vi "standard frame scan geometry_MD.vi"() -> (3 "frame scan geometry out":waveform(dbl)[](array[waveform]))   [LabVIEW 2012]
uses:
  GFG/GFGnumericGet.vi
  GFG/GFGbooleanGet.vi
  <vilib>/Analysis/coordinate.llb/2D Cartesian Coordinate Rotation (Array).vi
  GFG/GFG library.lvlib
  <vilib>/Analysis/NI_AALPro.lvlib
panel:
  out "x waveform":waveform(dbl)
  out "y waveform":waveform(dbl)
  out "Waveform Graph 2":waveform(dbl)(graph)
  out "Waveform Graph":waveform(dbl)(graph)
  out "y waveform (two frames)":dbl[](array[numeric])
  out "x waveform (two frames)":dbl[](array[numeric])
  out "XY Graph":cluster{"Y":dbl[], "Y":dbl[]}[](graph)
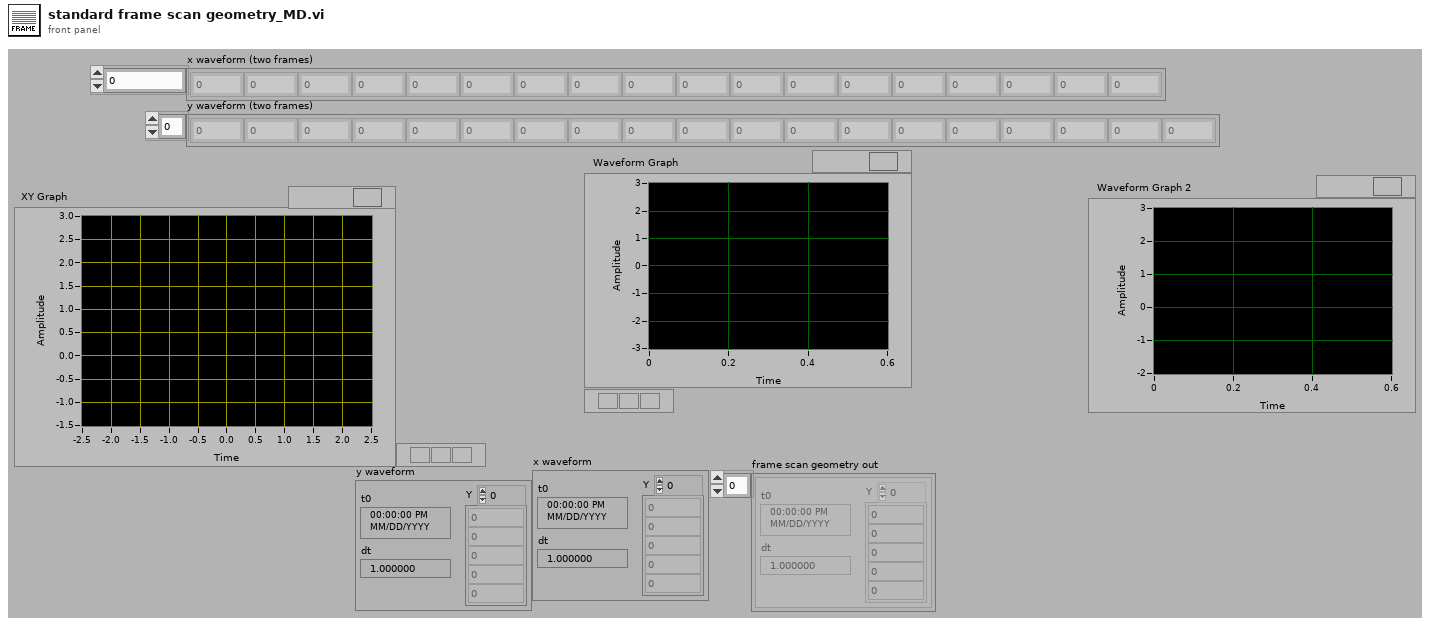
[diagram p1: front panel]
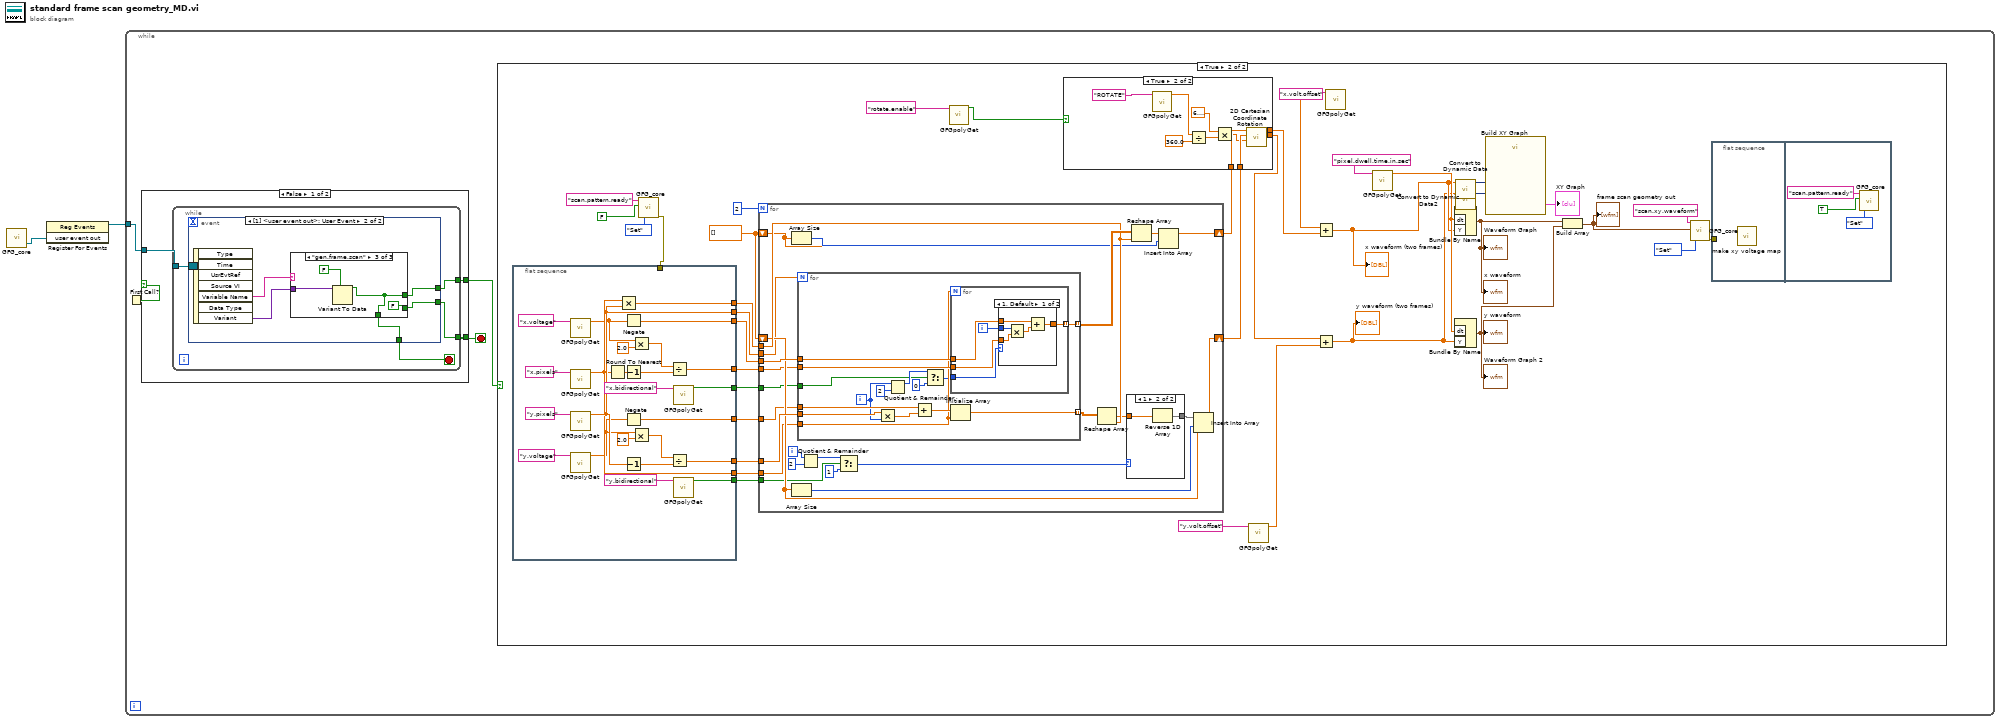
[diagram p0: block diagram]
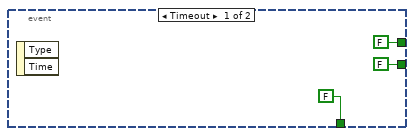
[diagram p2: hidden frame]
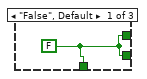
[diagram p3: hidden frame]
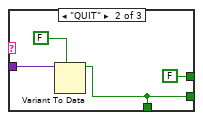
[diagram p4: hidden frame]
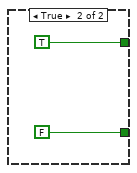
[diagram p5: hidden frame]
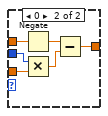
[diagram p9: hidden frame]
diagram:
  n1 = call "GFG_core.vi"() -> ("user event out"=w2:refnum<user-event>)  [unwired: 13 in, 6 out]
  n2 = register-events(w2) -> (reference out=w1:refnum<event-registration>)  [unwired: 2 in, 1 out]
  n3 = while {
    tunnel: w1 -> [w6]
    stop <- w5 stop-if-true
    n4 = First Call?() -> (First Call?: T/F=w3:bool)
    n5 = case shown="False" w3 {
      tunnel: w6 -> [w9 _]
      tunnel: [w8 FALSE ("NewVal")] -> w5
      tunnel: [w7 TRUE ("NewVal")] -> w4
      frame False {
        n6 = while {
          tunnel: w9 -> [w13]
          tunnel: [w11] -> w8
          tunnel: [w12] -> w7
          stop <- w10 stop-if-true
          n7 = event shown="[1] <user event out>: User Event" {
            selector: w13 -> [_ _]
            dyn-events: _ -> [_ _]
            timeout: _ -> [_ _]
            tunnel: [FALSE ("NewVal") w20] -> w12
            tunnel: [FALSE ("NewVal") w19] -> w11
            tunnel: [FALSE w17] -> w10
            event Timeout {
              n8 = event-data() -> ()  [unwired: 1 in, 2 out]
            }
            event User Event {
              n9 = event-data() -> ("Variable Name"=w21:string, "Variant"=w18:variant)  [unwired: 1 in, 5 out]
              n10 = case shown="\"gen.frame.scan\"" w21 {
                tunnel: [w22 FALSE ("NewVal") w27] -> w20
                tunnel: [w22 w23 FALSE] -> w19
                tunnel: w18 -> [_ w26 w28]
                tunnel: [w22 w23 w27] -> w17
                frame "False", Default {
                  w22 = FALSE ("NewVal")
                }
                frame "QUIT" {
                  n11 = Variant To Data(type=FALSE ("NewVal"), Variant=w26) -> (data=w23:bool)  [unwired: 1 in, 1 out]
                }
                frame "gen.frame.scan" {
                  n12 = Variant To Data(type=FALSE ("NewVal"), Variant=w28) -> (data=w27:bool)  [unwired: 1 in, 1 out]
                }
              }
            }
          }
        }
      }
      frame True {
      }
    }
    n13 = case shown="True" w4 {
      frame False {
      }
      frame True {
        w64 = dbl[] []
        n14 = flat-sequence {
          tunnel: [w92] -> w70
          tunnel: [w91] -> w69
          tunnel: [w89] -> w63
          tunnel: [w85] -> w62
          tunnel: [w84] -> w61
          tunnel: [w83] -> w60
          tunnel: [w81] -> w59
          tunnel: [w75] -> w58
          tunnel: [w73] -> w57
          tunnel: w33 -> [_]
          frame #0 {
            n15 = call-poly "GFGpolyGet.vi"("Variable Name in"="x.voltage" ("Tag in")) -> ("Numeric"=w79:dbl)  [unwired: 9 in, 1 out]
            n16 = call-poly "GFGpolyGet.vi"("Variable Name in"="x.pixels" ("Tag in")) -> ("Numeric"=w81:dbl)  [unwired: 9 in, 1 out]
            n17 = call-poly "GFGpolyGet.vi"("Variable Name in"="y.pixels" ("Tag in")) -> ("Numeric"=w83:dbl)  [unwired: 9 in, 1 out]
            n18 = call-poly "GFGpolyGet.vi"("Variable Name in"="y.voltage" ("Tag in")) -> ("Numeric"=w77:dbl)  [unwired: 9 in, 1 out]
            n19 = Round To Nearest(number=w81) -> (nearest integer value=w71:dbl)
            n20 = Multiply(x=w81, y=w83) -> (x*y=w84:dbl)
            n21 = Negate(x=w79) -> (-x=w92:dbl)
            n22 = Decrement(x=w71) -> (x-1=w88:dbl)
            n23 = Negate(x=w77) -> (-x=w89:dbl)
            n24 = Decrement(x=w83) -> (x-1=w90:dbl)
            n25 = Multiply(x=w79, y=2.0) -> (x*y=w87:dbl)
            n26 = Multiply(x=w77, y=2.0) -> (x*y=w93:dbl)
            n27 = Divide(x=w87, y=w88) -> (x/y=w85:dbl)
            n28 = Divide(x=w93, y=w90) -> (x/y=w91:dbl)
            n29 = call-poly "GFGpolyGet.vi"("Variable Name in"="x.bidirectional" ("Tag in")) -> ("Boolean"=w73:bool)  [unwired: 10 in]
            n30 = call-poly "GFGpolyGet.vi"("Variable Name in"="y.bidirectional" ("Tag in")) -> ("Boolean"=w75:bool)  [unwired: 10 in]
          }
        }
        n31 = call "GFG_core.vi"("Variable Name in"="scan.pattern.ready", "Variant in"=FALSE, "Action"=enum16{"Init", "Set", "Get"}."Set") -> ("error out"=w33:errorcluster)  [unwired: 10 in, 6 out]
        n32 = for {
          N: 2 -> [_]
          tunnel: w70 -> [w134]
          tunnel: w69 -> [w133]
          tunnel: w60 -> [w116]
          tunnel: w61 -> [w130]
          shift-right: [w124] -> w42
          shift-left: w64 -> [w126]
          shift-right: [w120] -> w41
          shift-left: w64 -> [w122]
          tunnel: w59 -> [w119]
          tunnel: w63 -> [w118]
          tunnel: w62 -> [w117]
          tunnel: w58 -> [w111]
          tunnel: w57 -> [w110]
          i -> [w129]
          n33 = Array Size(array=w126) -> (size(s)=w127:i32)
          n34 = Array Size(array=w122) -> (size(s)=w121:i32)
          n35 = for {
            N: w116 -> [_]
            tunnel: w119 -> [w144]
            tunnel: w134 -> [w146]
            tunnel: w133 -> [w152]
            tunnel: [w149] -> w132 mode=indexing
            tunnel: [w148] -> w131 mode=indexing
            tunnel: w118 -> [w147]
            tunnel: w117 -> [w145]
            tunnel: w110 -> [w138]
            i -> [w140]
            n36 = Multiply(x=w152, y=w140) -> (x*y=w151:dbl)
            n37 = Quotient & Remainder(x=w140, y=2) -> (x-y*floor(x/y)=w143:i32)  [unwired: 1 out]
            n38 = Add(x=w147, y=w151) -> (x+y=w150:dbl)
            n39 = Select(t=w143, s=w138, f=0) -> (s? t:f=w139:i32)
            n40 = for {
              N: w144 -> [_]
              tunnel: w145 -> [w157]
              tunnel: [w156] -> w149 mode=indexing
              tunnel: w146 -> [w155]
              tunnel: w139 -> [w153]
              i -> [w154]
              n41 = case shown="1, Default" w153 {
                tunnel: w157 -> [w162 w168]
                tunnel: [w161 w167] -> w156
                tunnel: w155 -> [w160 w166]
                tunnel: w154 -> [w158 w164]
                frame 1, Default {
                  n42 = Multiply(x=w158, y=w162) -> (x*y=w159:dbl)
                  n43 = Add(x=w160, y=w159) -> (x+y=w161:dbl)
                }
                frame 0 {
                  n44 = Negate(x=w166) -> (-x=w163:dbl)
                  n45 = Multiply(x=w164, y=w168) -> (x*y=w165:dbl)
                  n46 = Subtract(x=w163, y=w165) -> (x-y=w167:dbl)
                }
              }
            }
            n47 = Initialize Array(w150, w144) -> (w148:dbl[])
          }
          n48 = Quotient & Remainder(x=w129, y=2) -> (x-y*floor(x/y)=w113:i32)  [unwired: 1 out]
          n49 = Select(t=w113, s=w111, f=1) -> (s? t:f=w112:i32)
          n50 = Reshape Array(w131, w130) -> (w128:dbl[])
          n51 = case shown="1" w112 {
            tunnel: [w135 w136] -> w123
            tunnel: w128 -> [w135 w137]
            frame 0, Default {
            }
            frame 1 {
              n52 = Reverse 1D Array(array=w137) -> (reversed array=w136:dbl[])
            }
          }
          n53 = Reshape Array(w132, w130) -> (w125:dbl[])
          n54 = Insert Into Array(array=w125, index=w127, new element=w126) -> (w124:dbl[])
          n55 = Insert Into Array(array=w123, index=w121, new element=w122) -> (w120:dbl[])
        }
        n56 = call-poly "GFGpolyGet.vi"("Variable Name in"="rotate.enable" ("Tag in")) -> ("Boolean"=w44:bool)  [unwired: 10 in]
        n57 = case shown="True" w44 {
          tunnel: w42 -> [w98 w109]
          tunnel: w41 -> [w99 w108]
          tunnel: [w98 w101] -> w40
          tunnel: [w99 w100] -> w39
          frame False {
          }
          frame True {
            n58 = call-poly "GFGpolyGet.vi"("Variable Name in"="ROTATE" ("Tag in")) -> ("Numeric"=w103:dbl)  [unwired: 9 in, 1 out]
            n59 = Divide(x=w103, y=360.0) -> (x/y=w104:dbl)
            n60 = Multiply(x=6.283185307179586, y=w104) -> (x*y=w102:dbl)
            n61 = call-poly <vilib>:"2D Cartesian Coordinate Rotation.vi"("theta"=w102, "Y"=w108, "X"=w109) -> ("Y Out"=w100:dbl[], "X Out"=w101:dbl[])  [unwired: 6 in, 1 out]
          }
        }
        n62 = call-poly "GFGpolyGet.vi"("Variable Name in"="y.volt.offset" ("Tag in")) -> ("Numeric"=w52:dbl)  [unwired: 9 in, 1 out]
        n63 = Add(x=w39, y=w52) -> (x+y=w37:dbl[])
        "y waveform (two frames)" <- w37
        n64 = call-poly "GFGpolyGet.vi"("Variable Name in"="x.volt.offset" ("Tag in")) -> ("Numeric"=w54:dbl)  [unwired: 9 in, 1 out]
        n65 = Add(x=w54, y=w40) -> (x+y=w38:dbl[])
        "x waveform (two frames)" <- w38
        n66 = call-poly "GFGpolyGet.vi"("Variable Name in"="pixel.dwell.time.in.sec" ("Tag in")) -> ("Numeric"=w46:dbl)  [unwired: 9 in, 1 out]
        n67 = Bundle By Name("dt"=w46, "Y"=w38) -> (w51:waveform(dbl))  [unwired: 1 in]
        "Waveform Graph" <- w51
        "x waveform" <- w51
        n68 = Bundle By Name("dt"=w46, "Y"=w37) -> (w50:waveform(dbl))  [unwired: 1 in]
        "Waveform Graph 2" <- w50
        "y waveform" <- w50
        n69 = call "Convert to Dynamic Data"("Array"=w38) -> ("Dynamic Data Type"=w67:dynamicdata)  [unwired: 3 in]
        n70 = call "Convert to Dynamic Data2"("Array"=w37) -> ("Dynamic Data Type"=w66:dynamicdata)  [unwired: 3 in]
        n71 = call "Build XY Graph"("Y Input"=w66, "X Input"=w67) -> ("XY Graph"=→"XY Graph":cluster{"Y":dbl[], "Y":dbl[]}[])  [unwired: 8 in, 1 out]
        n72 = Build Array(w51, w50) -> (w48:waveform(dbl)[])
        "frame scan geometry out" <- w48
        n73 = call "GFG_core.vi"("Variable Name in"="scan.xy.waveform", "Variant in"=w48, "Action"=enum16{"Init", "Set", "Get"}."Set") -> ("error out"=w43:errorcluster)  [unwired: 10 in, 6 out]
        n74 = flat-sequence {
          tunnel: w43 -> [_]
          frame #0 {
            n75 = call "make xy voltage map.vi"() -> ()  [unwired: 12 in]
          }
          frame #1 {
            n76 = call "GFG_core.vi"("Variable Name in"="scan.pattern.ready", "Variant in"=TRUE, "Action"=enum16{"Init", "Set", "Get"}."Set") -> ()  [unwired: 10 in, 7 out]
          }
        }
      }
    }
  }
